vi "FTP_RemoveRemoteFile.vi"(5 "password":string, 7 "user":string="anonymous", 8 "error in":errorcluster, 10 "File Path":path, 11 "IP Address":string) -> (0 "error out":errorcluster)   [LabVIEW 2014, in "hse-network.lvlib"]
doc: "____\nHAMPEL SOFTWARE ENGINEERING v0.7.0 (2018-07-16 18:12)"
uses:
  hse-network.lvlib
  <vilib>/FTP/NI_FTP.lvlib
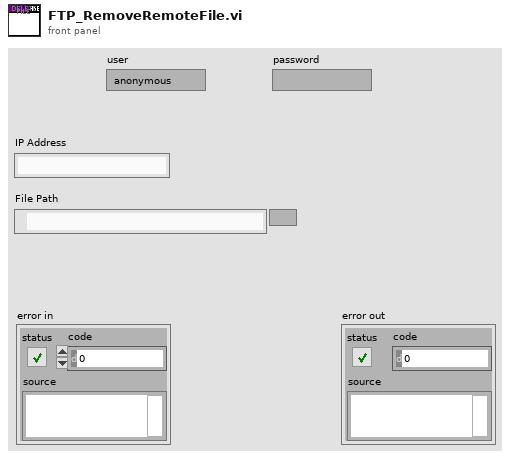
[diagram p1: front panel]
types:
  T1 = typedef "NI_FTP.lvlib/FTP Session.ctl" = refnum<k5>
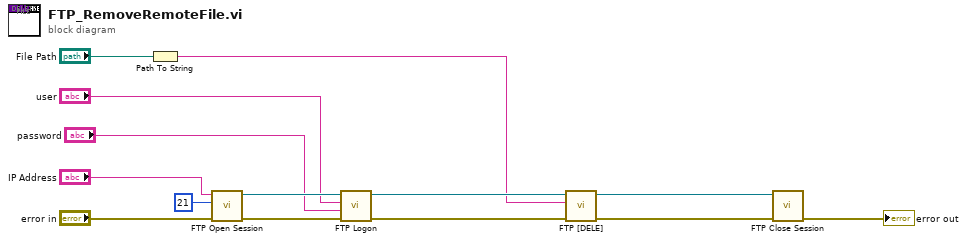
[diagram p0: block diagram]
diagram:
  n1 = Path To String(path="File Path") -> (string=w1:string)
  n2 = call <vilib>:"FTP Open Session.vi"("error in (no error)"="error in", "remote port (21)"=u16 21, "address"="IP Address") -> ("error out"=w9:errorcluster, "ftp session"=w8:T1)  [unwired: 5 in, 2 out]
  n3 = call <vilib>:"FTP Logon.vi"("error in (no error)"=w9, "password"="password", "user"="user", "ftp session"=w8) -> ("error out"=w5:errorcluster, "ftp session out"=w2:T1)  [unwired: 4 in, 2 out]
  n4 = call <vilib>:"FTP [DELE].vi"("error in (no error)"=w5, "file path"=w1, "ftp session"=w2) -> ("error out"=w4:errorcluster, "ftp session out"=w3:T1)  [unwired: 5 in, 2 out]
  n5 = call <vilib>:"FTP Close Session.vi"("error in (no error)"=w4, "ftp session"=w3) -> ("error out"=→"error out":errorcluster)  [unwired: 6 in, 3 out]
